vi "myRIO_BRig_FPGA_v3,52__PortC.vi"() -> ()   [LabVIEW 2014]
uses:
  <vilib>/rvi/Emulation/niFpgaGetClockAttributes.vi
  <vilib>/rvi/Emulation/niFpgaSctlEmulationGetInTimedLoop.vi
  <vilib>/rvi/Emulation/niFpgaEmulationReportErrorSimple.vi
  <vilib>/rvi/eio/common/nirviEmuTemplateMethod_errors.vi
  <vilib>/rvi/Emulation/niFpgaCriticalErrorInLSC.vi
  <vilib>/eio/EIONode/EIONode.xnode
panel:
  out "count_timeTrial":u32
  in  "timeTrial":bool
  in  "k1__counter_per_ms":u16=100 min=100 max=40000 step=1
  in  "laser_Nshutter":u32=100
  in  "AnaOut_0":i16
  in  "laser_Nvalley":u32=100
  in  "laser_Npeak":u32=100
  in  "laserledMTrig":bool
  in  "laser_selWro_Ntotal":u32=100
  in  "laser_selWro_NDelay":u32
  in  "laser_selRew_Ntotal":u32=100
  in  "laser_selRew_Ndelay":u32
  in  "laserResponse_reward_LED":bool
  in  "laserResponse_wrong_LED":bool
  out "SelectWrong":bool
  out "SelectReward":bool
  in  "laserResponse_wrong":bool
  in  "laserResponse_reward":bool
  in  "Left(F)_or_Right(T)":bool
  in  "ignoreWrong":bool
  in  "SelectionState":bool
  in  "laserMTrig":bool
  in  "FPGA_Stop":bool
  in  "audioTrigger_L":bool
  in  "audioTrigger_R":bool
  in  "audioFreq_L_kHz":u8=14 min=1 max=14 step=1
  in  "audioAmp_L":u16=1 min=1 max=32767 step=1
  in  "audioFreq_R_kHz":u8=14 min=1 max=14 step=1
  in  "audioAmp_R":u16=1 min=1 max=32767 step=1
  in  "A3_SL":bool
  in  "A1_SR":bool
  in  "Counts_Reset":bool
  out "A4_LickR":u32
  out "A2_LickL":u32
  in  "A6_Act":bool
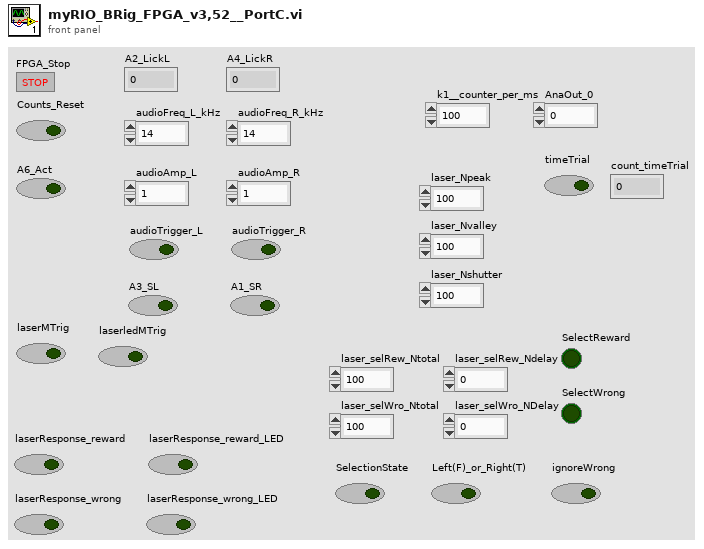
[diagram p1: front panel]
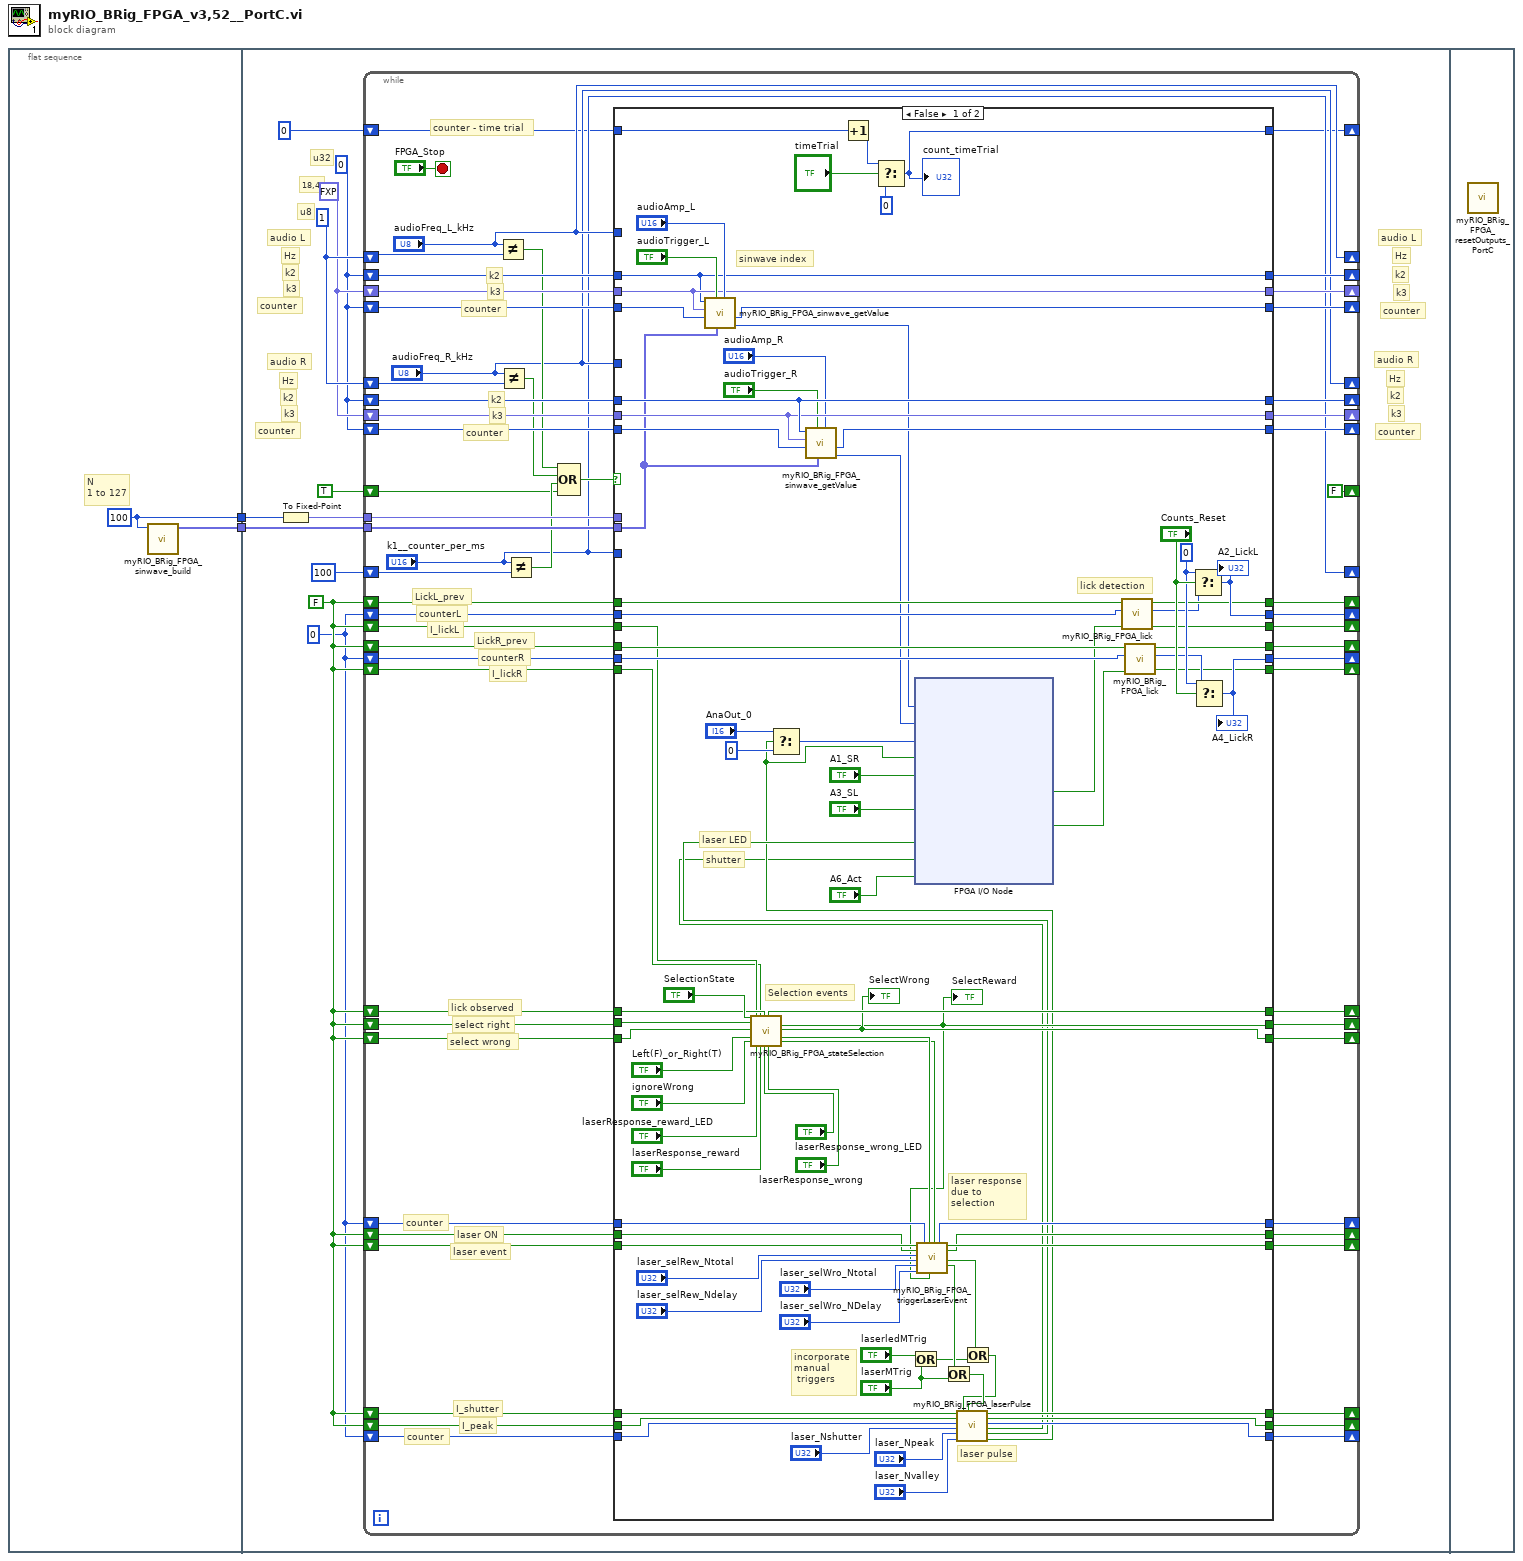
[diagram p0: block diagram]
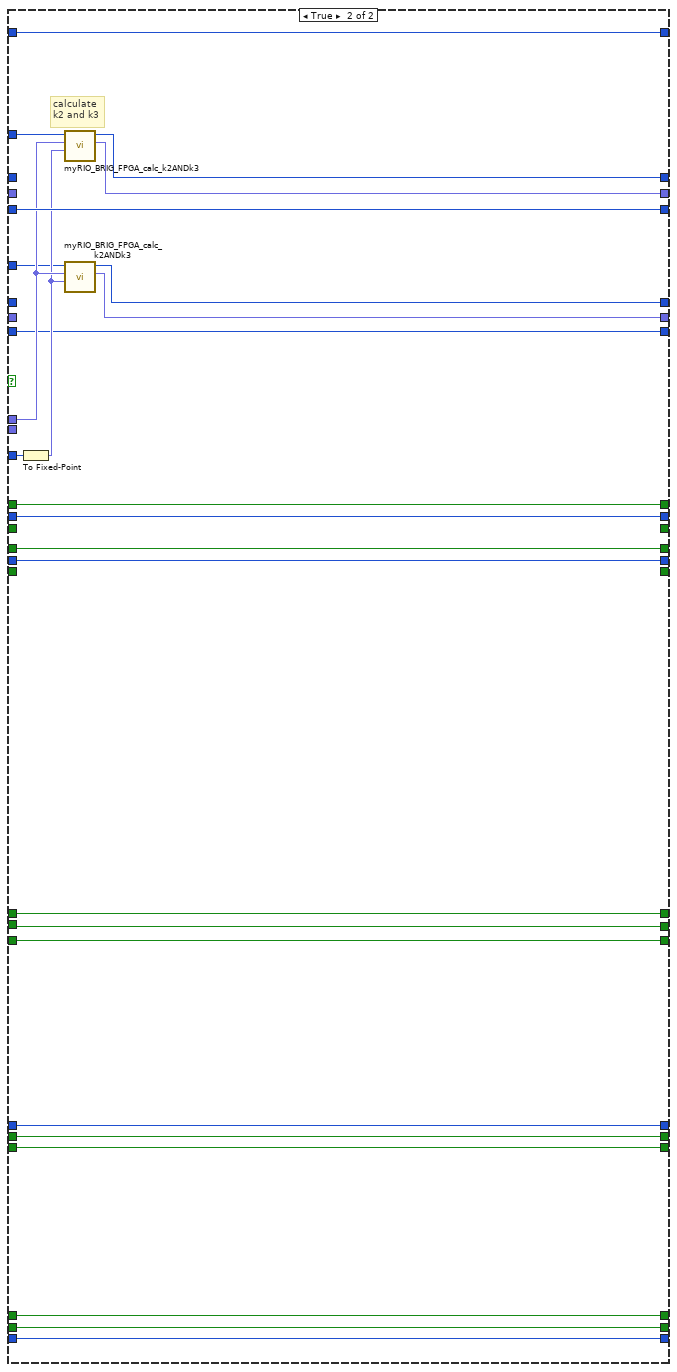
[diagram p2: hidden frame]
diagram:
  n1 = flat-sequence {
    tunnel: [w4] -> w2
    tunnel: [w3] -> w1
    tunnel: w2 -> [w15]
    tunnel: w1 -> [w14]
    frame #0 {
      w3 = 100 ("dimension size")
      # "N\n1 to 127"
      n2 = call "myRIO_BRig_FPGA_sinwave_build.vi"("input_Npts"=w3) -> ("output_array_sin"=w4:fxp<+/-,16,2>[])  [unwired: 10 in]
    }
    frame #1 {
      w6 = u32 0
      w7 = FALSE
      w10 = u32 0
      w11 = fxp<+,18,4> 0.0
      w12 = u8 1
      # "counter"
      # "k3"
      # "k2"
      # "counter"
      # "k3"
      # "k2"
      # "counter"
      # "counter"
      # "u32"
      # "k3"
      # "k2"
      # "k3"
      # "18,4"
      # "u8"
      # "Hz"
      # "Hz"
      # "audio R"
      # "audio L"
      # "Hz"
      # "k2"
      # "Hz"
      # "audio R"
      # "audio L"
      n3 = To Fixed-Point(number=w14) -> (fixed-point=w13:fxp<+,7,7>)  [unwired: 1 in]
      n4 = while {
        shift-right: ["audioFreq_L_kHz"] -> _
        shift-left: w12 -> [w74]
        shift-right: [w68] -> _
        shift-left: w10 -> [w72]
        shift-right: ["audioFreq_R_kHz"] -> _
        shift-left: w12 -> [w64]
        tunnel: w15 -> [w71]
        tunnel: w13 -> [w70]
        shift-right: [w67] -> _
        shift-left: w11 -> [w69]
        shift-right: [w65] -> _
        shift-left: w10 -> [w66]
        shift-right: [w62] -> _
        shift-left: w10 -> [w63]
        shift-right: [w60] -> _
        shift-left: w11 -> [w61]
        shift-right: [w58] -> _
        shift-left: w10 -> [w59]
        shift-right: ["k1__counter_per_ms"] -> _
        shift-left: u16 100 ("y") -> [w57]
        shift-right: [FALSE] -> _
        shift-left: TRUE -> [w52]
        shift-right: [w45] -> _
        shift-left: w7 -> [w47]
        shift-right: [w44] -> _
        shift-left: w7 -> [w46]
        shift-right: [w42] -> _
        shift-left: w6 -> [w43]
        shift-right: [w40] -> _
        shift-left: w6 -> [w41]
        shift-right: [w38] -> _
        shift-left: w7 -> [w39]
        shift-right: [w35] -> _
        shift-left: w7 -> [w37]
        shift-right: [w34] -> _
        shift-left: w7 -> [w36]
        shift-right: [w31] -> _
        shift-left: w7 -> [w30]
        shift-right: [w32] -> _
        shift-left: w7 -> [w33]
        shift-right: [w28] -> _
        shift-left: w6 -> [w29]
        shift-right: [w24] -> _
        shift-left: w7 -> [w27]
        shift-right: [w23] -> _
        shift-left: w7 -> [w26]
        shift-right: [w22] -> _
        shift-left: w6 -> [w25]
        shift-right: [w20] -> _
        shift-left: w7 -> [w21]
        shift-right: [w18] -> _
        shift-left: w7 -> [w19]
        shift-right: [w16] -> _
        shift-left: u32 0 -> [w17]
        stop <- "FPGA_Stop" stop-if-true
        # "counter"
        # "k3"
        # "k2"
        # "counter"
        # "k3"
        # "k2"
        # "counter - time trial"
        # "counter"
        # "counter"
        # "I_lickR"
        # "counterR"
        # "LickR_prev"
        # "I_lickL"
        # "counterL"
        # "LickL_prev"
        # "I_shutter"
        # "I_peak"
        # "laser ON"
        # "laser event"
        # "select wrong"
        # "select right"
        # "lick observed"
        n5 = Not Equal?(x="audioFreq_L_kHz", y=w74) -> (x != y?=w56:bool)
        n6 = Not Equal?(x="audioFreq_R_kHz", y=w64) -> (x != y?=w55:bool)
        n7 = Not Equal?(x="k1__counter_per_ms", y=w57) -> (x != y?=w53:bool)
        n8 = Compound Arithmetic op=OR(w56, w55, w53, w52) -> (w54:bool)
        n9 = case shown="False" w54 {
          tunnel: w72 -> [w128 _]
          tunnel: "audioFreq_L_kHz" -> [_ w186]
          tunnel: w71 -> [w121 _]
          tunnel: w70 -> [_ w182]
          tunnel: "k1__counter_per_ms" -> [_ w187]
          tunnel: w69 -> [w129 _]
          tunnel: [w128 w185] -> w68
          tunnel: [w129 w184] -> w67
          tunnel: w66 -> [w133 w183]
          tunnel: [w130 w183] -> w65
          tunnel: w63 -> [w125 _]
          tunnel: [w125 w178] -> w62
          tunnel: w61 -> [w124 _]
          tunnel: [w124 w179] -> w60
          tunnel: w59 -> [w127 w177]
          tunnel: "audioFreq_R_kHz" -> [_ w180]
          tunnel: [w126 w177] -> w58
          tunnel: w47 -> [w116 w176]
          tunnel: w46 -> [w115 w175]
          tunnel: [w120 w176] -> w45
          tunnel: [w113 w175] -> w44
          tunnel: w43 -> [w117 w174]
          tunnel: [w162 w174] -> w42
          tunnel: w41 -> [w114 w173]
          tunnel: [w159 w173] -> w40
          tunnel: w39 -> [w155 w172]
          tunnel: [w154 w172] -> w38
          tunnel: w37 -> [w157 w171]
          tunnel: w36 -> [w156 w170]
          tunnel: [w106 w171] -> w35
          tunnel: [w147 w170] -> w34
          tunnel: w33 -> [w145 w169]
          tunnel: [w141 w169] -> w32
          tunnel: [w142 w168] -> w31
          tunnel: w30 -> [w146 w168]
          tunnel: w29 -> [w144 w167]
          tunnel: [w143 w167] -> w28
          tunnel: w27 -> [w100 w166]
          tunnel: w26 -> [w101 w165]
          tunnel: w25 -> [w102 w164]
          tunnel: [w103 w166] -> w24
          tunnel: [w104 w165] -> w23
          tunnel: [w105 w164] -> w22
          tunnel: w21 -> [w110 _]
          tunnel: [w119 _] -> w20
          tunnel: w19 -> [w109 _]
          tunnel: [w111 _] -> w18
          tunnel: w17 -> [w90 w163]
          tunnel: [w87 w163] -> w16
          frame False {
            w160 = u32 0 ("t")
            # "sinwave index"
            # "lick detection"
            # "laser pulse"
            # "incorporate\nmanual\n triggers"
            # "laser response\ndue to\nselection"
            # "Selection events"
            # "laser LED"
            # "shutter"
            n10 = call "myRIO_BRig_FPGA_sinwave_getValue.vi"("audioAmp"="audioAmp_L", "sinwave"=w121, "audioTrigger"="audioTrigger_L", "counter"=w133, "k3"=w129, "k2"=w128) -> ("output_audioValue"=w85:i16, "output_counter"=w130:u32)  [unwired: 4 in]
            n11 = call "myRIO_BRig_FPGA_stateSelection.vi"("I_selectionState"="SelectionState", "I_selectRight"=w157, "I_selectWrong"=w156, "I_Left(F)_or_Right(T)"="Left(F)_or_Right(T)", "I_ignoreWrong"="ignoreWrong", "I_lickL"=w110, "I_laserEvent_Reward"="laserResponse_reward_LED", "I_lickR"=w109, "I_laser_Reward"="laserResponse_reward", "I_lickObserved"=w155, "I_laserEvent_Wrong"="laserResponse_wrong_LED", "I_laser_Wrong"="laserResponse_wrong") -> ("output_I_lickObserved"=w154:bool, "output__I_selectRight"=w106:bool, "output__I_selectWrong"=w147:bool, "output_I_startLaserEvent"=w108:bool, "output_I_startLaser"=w107:bool)  [unwired: 11 in]
            "SelectWrong" <- w147
            "SelectReward" <- w106
            n12 = call "myRIO_BRig_FPGA_sinwave_getValue.vi"("audioAmp"="audioAmp_R", "sinwave"=w121, "audioTrigger"="audioTrigger_R", "counter"=w127, "k3"=w124, "k2"=w125) -> ("output_audioValue"=w84:i16, "output_counter"=w126:u32)  [unwired: 4 in]
            n13 = Increment(x=w90) -> (x+1=w89:u32)
            n14 = Select(t=w89, s="timeTrial", f=u32 0) -> (s? t:f=w87:u32)
            "count_timeTrial" <- w87
            n15 = Or(x="laserledMTrig", y="laserMTrig") -> (x .or. y?=w94:bool)
            n16 = call "myRIO_BRig_FPGA_triggerLaserEvent.vi"("I_laserEvent"=w146, "I_laser"=w145, "laser_selRew_Ntotal"="laser_selRew_Ntotal", "laser_selRew_Ndelay"="laser_selRew_Ndelay", "laser_selWro_Ntotal"="laser_selWro_Ntotal", "laser_selWro_NDelay"="laser_selWro_NDelay", "counter"=w144, "I_startLaserEvent"=w108, "selectReward"=w106, "I_startLaser"=w107) -> ("output_counter"=w143:u32, "output_I_laserEvent"=w142:bool, "output_I_laser"=w141:bool, "output_I_trigLaserEvent"=w96:bool, "output_I_trigLaser"=w95:bool)  [unwired: 5 in]
            n17 = Or(x=w95, y="laserMTrig") -> (x .or. y?=w92:bool)
            n18 = Or(x=w96, y=w94) -> (x .or. y?=w91:bool)
            n19 = call "myRIO_BRig_FPGA_laserPulse.vi"("I_shutter"=w100, "I_peak"=w101, "count"=w102, "laser_Nshutter"="laser_Nshutter", "laser_Npeak"="laser_Npeak", "laser_Nvalley"="laser_Nvalley", "I_laserEvent"=w91, "I_laser"=w92) -> ("output_I_shutter"=w103:bool, "output_I_peak"=w104:bool, "output_count"=w105:u32, "output_shutter"=w75:bool, "output_led"=w77:bool, "output_laser"=w76:bool)  [unwired: 6 in]
            n20 = Select(t="AnaOut_0", s=w76, f=i16 0) -> (s? t:f=w80:i16)
            n21 = xnode "FPGA I/O Node"("AudioOut/Left"=w85, "AudioOut/Right"=w84, "ConnectorC/AO0"=w80, "ConnectorC/DIO0"=w76, "ConnectorC/DIO1"="A1_SR", "ConnectorC/DIO3"="A3_SL", "ConnectorC/DIO5"=w77, "ConnectorC/DIO6"=w75, "ConnectorC/DIO7"="A6_Act") -> ("ConnectorC/DIO2"=w83:bool, "ConnectorC/DIO4"=w82:bool)  [unwired: 11 in, 11 out]
            n22 = call "myRIO_BRig_FPGA_lick.vi"("I_stateDetector_new"=w83, "counter"=w117, "I_stateDetector_prev"=w116) -> ("output_I_lick"=w119:bool, "output_counter"=w118:u32, "output_I_stateDetector_prev"=w120:bool)  [unwired: 6 in]
            n23 = call "myRIO_BRig_FPGA_lick.vi"("I_stateDetector_new"=w82, "counter"=w114, "I_stateDetector_prev"=w115) -> ("output_I_lick"=w111:bool, "output_counter"=w112:u32, "output_I_stateDetector_prev"=w113:bool)  [unwired: 6 in]
            n24 = Select(t=w160, s="Counts_Reset", f=w118) -> (s? t:f=w162:u32)
            "A2_LickL" <- w162
            n25 = Select(t=w160, s="Counts_Reset", f=w112) -> (s? t:f=w159:u32)
            "A4_LickR" <- w159
          }
          frame True {
            # "calculate\nk2 and k3"
            n26 = To Fixed-Point(number=w187) -> (fixed-point=w181:fxp<+,16,16>)  [unwired: 1 in]
            n27 = call "myRIO_BRIG_FPGA_calc_k2ANDk3.vi"("input_k1[count/ms]"=w181, "input_Npts"=w182, "input_freq[kHz]"=w186) -> ("output_k3"=w184:fxp<+,18,4>, "output_k2"=w185:u32)  [unwired: 7 in]
            n28 = call "myRIO_BRIG_FPGA_calc_k2ANDk3.vi"("input_k1[count/ms]"=w181, "input_Npts"=w182, "input_freq[kHz]"=w180) -> ("output_k3"=w179:fxp<+,18,4>, "output_k2"=w178:u32)  [unwired: 7 in]
          }
        }
      }
    }
    frame #2 {
      n29 = call "myRIO_BRig_FPGA_resetOutputs_PortC.vi"() -> ()  [unwired: 12 in]
    }
  }
